vi "Lechman_Target_A_2.vi"   [LabVIEW 2019]
uses:
  <vilib>/Platform/TimedLoop/XDataNode/timing_clust.ctl
  <vilib>/Platform/TimedLoop/XDataNode/nitl_modes.ctl
  <vilib>/Platform/TimedLoop/XDataNode/wakeup.ctl
  <vilib>/Platform/TimedLoop/XDataNode/XDataNode.xnode
  <vilib>/Platform/TimedLoop/XDataNode/XDNodeRunTimeDep.lvlib
  <resource>/objmgr/ni.dex.rc
types:
  T1 = typedef "XDNodeRunTimeDep.lvlib/timing_clust.ctl" = cluster{"Expected End [f-1]":u64, "Actual End [f-1]":u64, "Finished Late? [f-1]":bool, "Expected End [i-1]":u64, "Actual End [i-1]":u64, "Finished Late? [i-1]":bool, "Expected Start [i]":u64, "Actual Start [i]":u64, "Expected Start [f]":u64, "Actual Start [f]":u64, "Source Name":string, "Structure Name":string, "Period":i64, "Deadline":i64, "Offset":i64, "Start":i64, "Priority":i32, "Timeout":i32, "Mode":T2, "Wakeup Reason":T3, "Error":errorcluster, "Source Type":string, "Secondary Source Type":string, "Global End Time":u64, "Global Start Time":u64, "Frame Duration":u64, "Iteration Duration":u64, "Assigned CPU":i32, "I/O Scan Engine Mode":u32}
  T2 = typedef "XDNodeRunTimeDep.lvlib/nitl_modes.ctl" = enum32{"No Change", "Process missed periods, maintain original phase", "Discard missed periods, maintain original phase", "Process missed periods, ignore original phase", "Discard missed periods, ignore original phase"}
  T3 = typedef "XDNodeRunTimeDep.lvlib/wakeup.ctl" = enum32{"Normal", "Aborted", "Asynchronous wakeup", "Timing source error", "Timed loop error", "Timeout"}
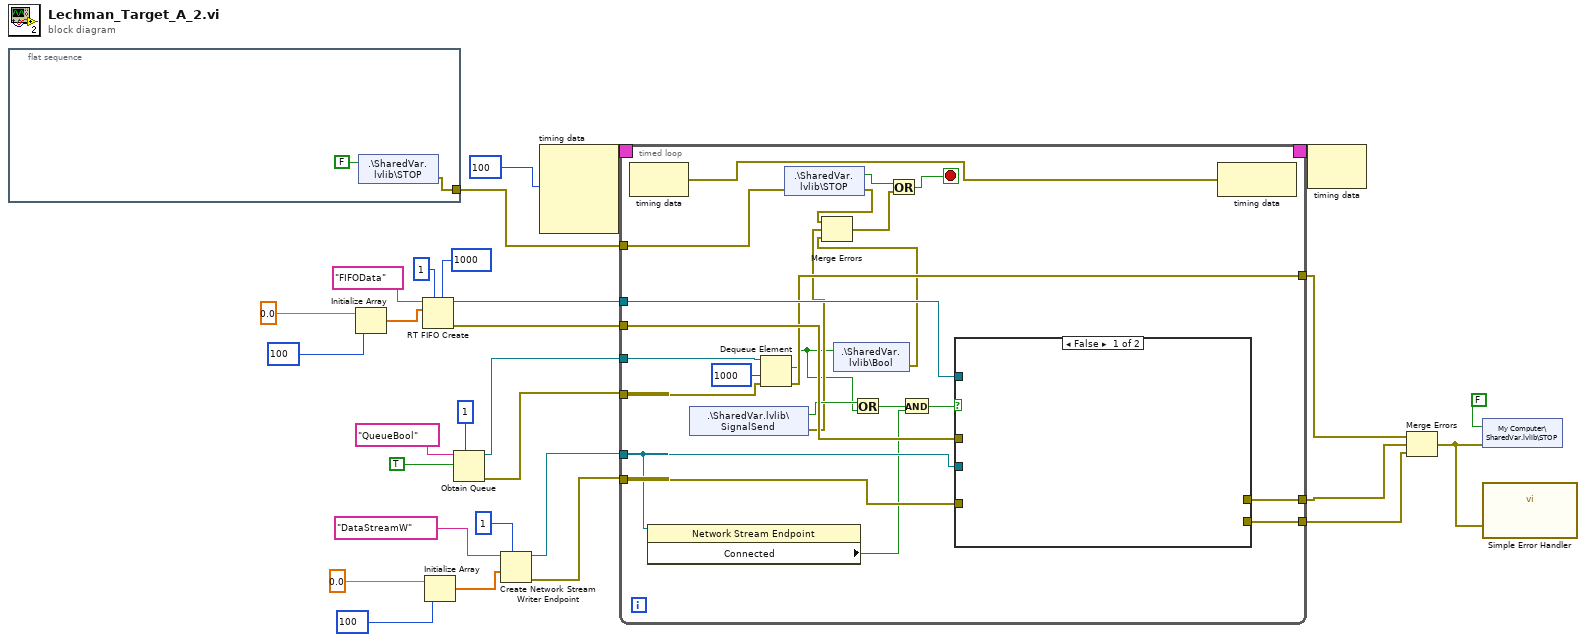
[diagram p0: block diagram]
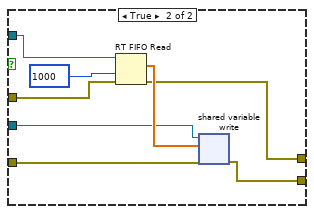
[diagram p2: hidden frame]
diagram:
  n1 = flat-sequence {
    tunnel: [w30] -> w7
    frame #0 {
      n2 = shared-variable ".\\SharedVar.lvlib\\STOP"(FALSE ("STOP")) -> (error out=w30:errorcluster)  [unwired: 1 in]
    }
  }
  n3 = Initialize Array(0.0, 100 ("dimension size")) -> (w23:dbl[])
  n4 = RT FIFO Create(0:"FIFOData" ("name (unnamed)"), 1:w23, 4:u32 1 ("size (10)"), 6:u32 1000 ("elements in array (1)")) -> (8:w6:refnum<k33>, 11:w10:errorcluster)  [unwired: 4 in, 1 out]
  n5 = Initialize Array(0.0, 100 ("dimension size")) -> (w15:dbl[])
  n6 = Obtain Queue(max queue size (-1, unlimited)=1, name (unnamed)="QueueBool", element data type=TRUE) -> (queue out=w12:refnum<queue>, error out=w9:errorcluster)  [unwired: 2 in, 1 out]
  n7 = Create Network Stream Writer Endpoint(7:1 ("writer buffer size"), 9:w15, 11:"DataStreamW" ("writer name")) -> (0:w8:errorcluster, 3:w11:refnum<k21>)  [unwired: 4 in]
  n8 = node-c288(i64 100 ("Period")) -> (w29:T1)  [unwired: 3 in]
  n9 = timed-loop {
    timing: w29 -> [_]
    timing-out: [_] -> w28
    tunnel: w12 -> [w53]
    tunnel: w11 -> [w38]
    tunnel: w10 -> [w52]
    tunnel: w9 -> [w51]
    tunnel: w8 -> [w45]
    tunnel: w7 -> [w50]
    tunnel: w6 -> [w46]
    tunnel: [w44] -> w3
    tunnel: [w43] -> w2
    tunnel: [w42] -> w1
    stop <- w49 stop-if-true
    n10 = node-c288() -> (w32:errorcluster)  [unwired: 1 in]
    n11 = property class="Network Stream Endpoint"(reference=w38) -> ("Connected"=w37:bool)  [unwired: 1 in, 2 out]
    n12 = shared-variable ".\\SharedVar.lvlib\\SignalSend"() -> (w39:bool, error out=w34:errorcluster)  [unwired: 1 in]
    n13 = Dequeue Element(queue=w53, timeout in ms (-1)=1000, error in (no error)=w51) -> (element=w33:bool, error out=w42:errorcluster)  [unwired: 2 out]
    n14 = shared-variable ".\\SharedVar.lvlib\\STOP"(error in=w50) -> (w48:bool, error out=w36:errorcluster)
    n15 = shared-variable ".\\SharedVar.lvlib\\Bool"(w33) -> (error out=w35:errorcluster)  [unwired: 1 in]
    n16 = Merge Errors(w36, w34, w35) -> (w47:errorcluster)
    n17 = Or(x=w39, y=w33) -> (x .or. y?=w41:bool)
    n18 = Or(x=w48, y=w47) -> (x .or. y?=w49:bool)
    n19 = And(x=w41, y=w37) -> (x .and. y?=w40:bool)
    n20 = case shown="False" w40 {
      tunnel: w52 -> [_ w61]
      tunnel: w45 -> [_ w60]
      tunnel: w46 -> [_ w59]
      tunnel: [_ w57] -> w44
      tunnel: [_ w56] -> w43
      tunnel: w38 -> [_ w55]
      frame False {
      }
      frame True {
        n21 = RT FIFO Read(0:w59, 2:1000 ("timeout in ms (0)"), 3:w61) -> (9:w58:dbl[], 11:w56:errorcluster)  [unwired: 1 in, 3 out]
        n22 = shared-variable-write(w55, w60, w58) -> (w57:errorcluster)  [unwired: 1 in, 2 out]
      }
    }
    n23 = node-c288(w32) -> ()  [unwired: 1 out]
  }
  n24 = node-c288(w28) -> ()  [unwired: 1 out]
  n25 = Merge Errors(w1, w2, w3) -> (w4:errorcluster)
  n26 = shared-variable "My Computer\\SharedVar.lvlib\\STOP"(FALSE ("STOP"), error in=w4) -> ()  [unwired: 1 out]
  n27 = call <vilib>:"Simple Error Handler.vi"("error in (no error)"=w4) -> ()  [unwired: 4 in, 5 out]
